vi "GetMSGName.vi"(11 "Incriment Msg in":refnum<class "Incriment Msg.lvclass">) -> (2 "NAME":string, 3 "Incriment Msg out":refnum<class "Incriment Msg.lvclass">)   [LabVIEW 2020, in "Test-Client.lvlib" / "Incriment Msg.lvclass"]
uses:
  Incriment Msg.lvclass
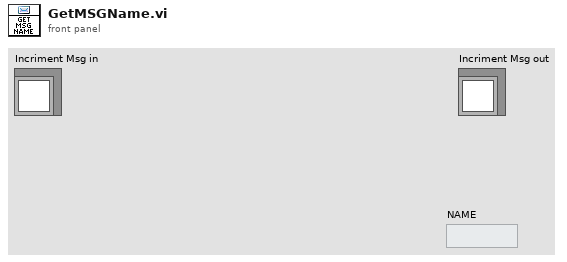
[diagram p1: front panel]
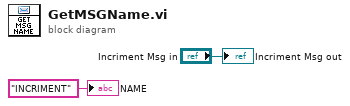
[diagram p0: block diagram]
diagram:
  "Incriment Msg out" <- "Incriment Msg in"
  "NAME" <- "INCRIMENT" ("NAME")
